vi "DutyAccelM2.vi"() -> ()   [LabVIEW 2015]
uses:
  <instrlib>/Ion Motion Roboclaw/Ion Motion Roboclaw.lvlib
panel:
  in  "Address":u8
  in  "stop":bool
  in  "Accel":u32(slide) max=655360 step=1000 scale=0.0..655360.0
  in  "Duty":i32(slide)=-32767 min=-32767 max=32767 step=100 scale=-32767.0..32767.0
  out "Valid":bool
  out "error out":errorcluster
  in  "COM port":refnum<visa-resource-name>
  in  "baud rate (38400)":u32
  in  "error in (no error)":errorcluster
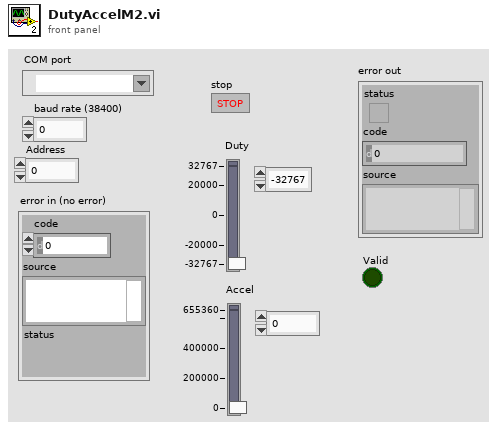
[diagram p1: front panel]
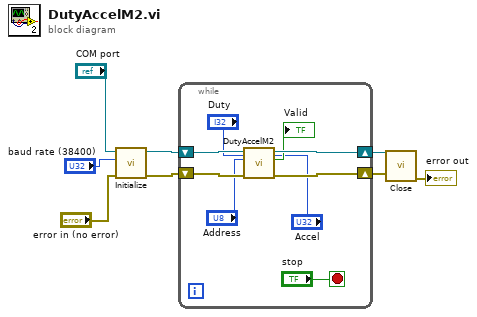
[diagram p0: block diagram]
diagram:
  n1 = call <instrlib>:"Initialize.vi"("error in (no error)"="error in (no error)", "baud rate (38400)"="baud rate (38400)", "COM port"="COM port") -> ("error out"=w7:errorcluster, "VISA resource name out"=w8:refnum<visa-resource-name>)  [unwired: 7 in]
  n2 = while {
    shift-right: [w15] -> w6
    shift-left: w8 -> [w17]
    shift-right: [w14] -> w5
    shift-left: w7 -> [w16]
    stop <- "stop" stop-if-true
    n3 = call <instrlib>:"DutyAccelM2.vi"("Accel"="Accel", "Duty"="Duty", "error in (no error)"=w16, "Address"="Address", "VISA Refnum in"=w17) -> ("error out"=w14:errorcluster, "Valid"=→"Valid":bool, "VISA Refnum out"=w15:refnum<visa-resource-name>)  [unwired: 4 in]
  }
  n4 = call <instrlib>:"Close.vi"("error in (no error)"=w5, "VISA resource name"=w6) -> ("error out"=→"error out":errorcluster)  [unwired: 9 in]
